vi "Goto RGB Color Now.vi"() -> ()   [LabVIEW 2013]
uses:
  <vilib>/LabVIEW Hacker/LINX/Private/Device/Type Defs/TCP Config.ctl
  <vilib>/LabVIEW Hacker/LINX/Private/Type Defs/Interface.ctl
  <vilib>/LabVIEW Hacker/LINX/Public/Sensors/BlinkM/BlinkM.lvlib
  <vilib>/LabVIEW Hacker/LINX/LVH-LINX.lvlib
  <vilib>/ptbypt/NI_PtbyPt.lvlib
  <vilib>/LabVIEW Hacker/LINX/Private/Device/Device.lvlib
panel:
  out "Loop Time":dbl format="%0.2f"
  in  "Stop Button":bool
  out "Error Out":errorcluster={"status"=TRUE, "code"=1, "source"="Property Node (arg 1) in VISA Configure Serial Port (Instr).vi->LVH-LINX.lvlib:Device.lvlib:Serial Open.vi->LVH-LINX.lvlib:Device.lvlib:Initialize Device.vi->LVH-LINX.lvlib:Initialize.vi->Goto RGB Color Now.vi"}
  in  "Color":u32(colorbox)
  in  "Interface":T1=enum."TCP"
  in  "Serial Port":refnum<visa-resource-name>="COM7"
  in  "TCP Configuration":T2={"IP Address"="10.2.106.213", "Port"=6921}
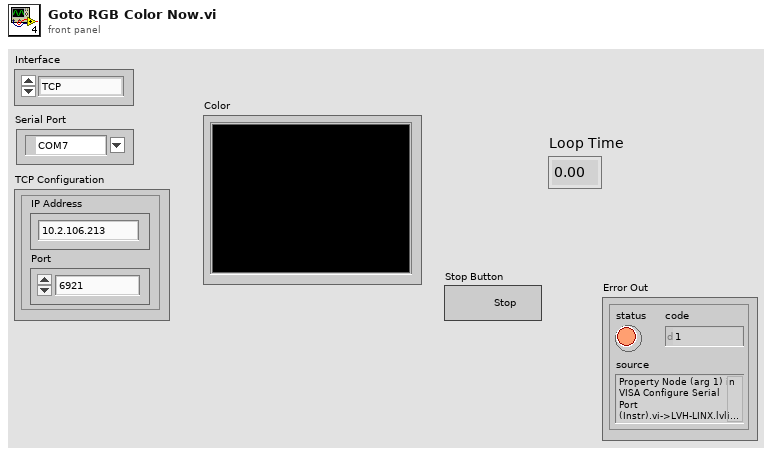
[diagram p1: front panel]
types:
  T1 = typedef "LVH-LINX.lvlib/Interface.ctl" = enum16{"Serial", "TCP"}
  T2 = typedef "LVH-LINX.lvlib/Device.lvlib/TCP Config.ctl" = cluster{"IP Address":string, "Port":u16}
  T3 = typedef "LVH-LINX.lvlib/LINX Ref.ctl" = cluster{"Platform":T4, "Interface":T1, "LINX Device Config":T5}
  T4 = typedef "LVH-LINX.lvlib/Platform.ctl" = enum16{"LINX", "myRIO"}
  T5 = typedef "LVH-LINX.lvlib/Device.lvlib/LINX Device Config.ctl" = cluster{"Interface":T1, "COM Port":refnum<visa-resource-name>, "TCP Configuration":T2, "Device Family":T6, "Device ID":u8, "Device Name":string, "TCP Ref":refnum<k5>}
  T6 = typedef "LVH-LINX.lvlib/Device Family.ctl" = enum8{"National Instruments", "Digilent", "Arduino"}
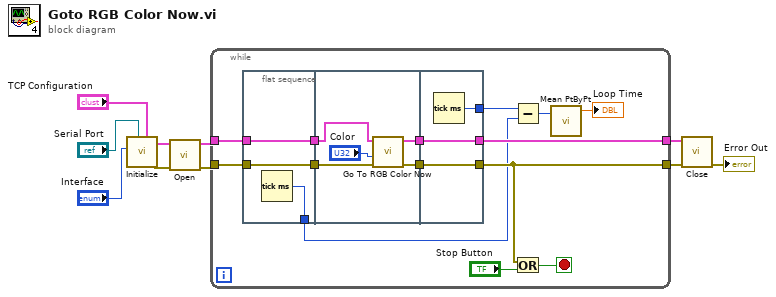
[diagram p0: block diagram]
diagram:
  n1 = call <vilib>:"Initialize.vi"("TCP Configuration"="TCP Configuration", "Serial Port"="Serial Port", "Interface"="Interface") -> ("Error Out"=w1:errorcluster, "LINX Ref"=w4:T3)  [unwired: 6 in, 1 out]
  n2 = call <vilib>:"Open.vi"("Error In"=w1, "LINX Resource"=w4) -> ("Error Out"=w2:errorcluster, "LINX Resource"=w3:T3)  [unwired: 8 in]
  n3 = while {
    tunnel: w3 -> [w24]
    tunnel: w2 -> [w23]
    tunnel: [w19] -> w6
    tunnel: [w22] -> w5
    stop <- w21 stop-if-true
    n4 = flat-sequence {
      tunnel: w23 -> [w26]
      tunnel: w24 -> [w27]
      tunnel: [w27] -> w16
      tunnel: [w26] -> w15
      tunnel: [w25] -> w14
      tunnel: [w29] -> w18
      tunnel: [w28] -> w17
      tunnel: w16 -> [w31]
      tunnel: w15 -> [w30]
      tunnel: [w34] -> w19
      tunnel: [w35] -> w22
      tunnel: w18 -> [w35]
      tunnel: w17 -> [w34]
      tunnel: [w33] -> w13
      frame #0 {
        n5 = Tick Count (ms)() -> (millisecond timer value=w25:u32)
      }
      frame #1 {
        n6 = call <vilib>:"Go To RGB Color Now.vi"("Error In"=w30, "Color"="Color", "LINX Resource"=w31) -> ("Error Out"=w28:errorcluster, "LINX Resource"=w29:T3)  [unwired: 7 in]
      }
      frame #2 {
        n7 = Tick Count (ms)() -> (millisecond timer value=w33:u32)
      }
    }
    n8 = Subtract(x=w13, y=w14) -> (x-y=w12:u32)
    n9 = Or(x=w19, y="Stop Button") -> (x .or. y?=w21:bool)
    n10 = call <vilib>:"Mean PtByPt.vi"("x"=w12) -> ("mean"=→"Loop Time":dbl)  [unwired: 3 in, 1 out]
  }
  n11 = call <vilib>:"Close.vi"("Error In"=w6, "LINX Resource"=w5) -> ("Error Out"=→"Error Out":errorcluster)  [unwired: 8 in, 1 out]
